vi "DAQmx Create CI Channel (sub).vi"(0 "task in":refnum<k21>, 1 "virtual channel name":string, 5 "physical channel name":tag, 7 "measurement type":i32(ring)=10125 items=["count events"=10125, "frequency"=10179, "period"=10256, "pulse width"=10359, "semi period"=10289, "pulse frequency"=15864, "pulse time"=15865, "pulse ticks"=15866, "two edge separation"=10267, "angular encoder"=10360, "linear encoder"=10361, "gps timestamp"=10362], 11 "error in":errorcluster, 13 "custom scale":tag) -> (4 "task out":refnum<k21>, 6 "channel names":string, 15 "error out":errorcluster)   [LabVIEW 2013]
uses:
  nilvaiu.dll
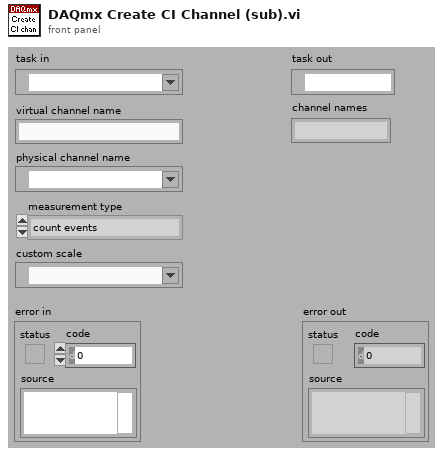
[diagram p1: front panel]
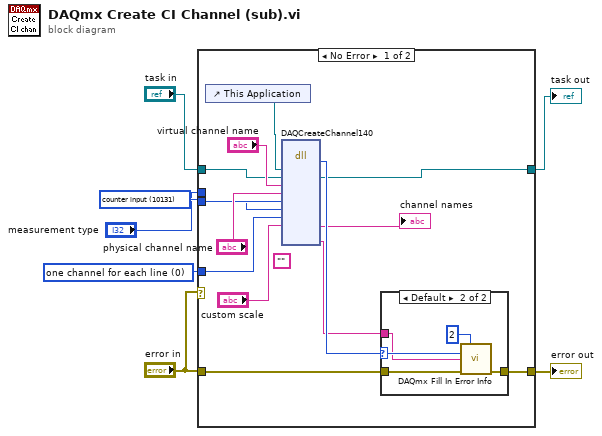
[diagram p0: block diagram]
diagram:
  w3 = 0 items=["one channel for each line", "one channel for all lines"] ("line grouping")
  w4 = 10131 items=["analog input"=10100, "analog output"=10102, "digital input"=10151, "digital output"=10153, "counter input"=10131, "counter output"=10132] ("channel type")
  n1 = case shown="No Error" "error in" {
    tunnel: [w17 w29] -> w7
    tunnel: "error in" -> [w19 w29]
    tunnel: "task in" -> [w9 w28]
    tunnel: "measurement type" -> [w16 _]
    tunnel: w4 -> [w15 _]
    tunnel: w3 -> [w11 _]
    tunnel: [w10 w28] -> w1
    frame No Error {
      (unwired) ""
      n2 = control-ref of="This Application"() -> (w8:refnum<vi>)
      n3 = dll-call lib="nilvaiu.*" fn="DAQCreateChannel140"("lvAppReference"=w8, "taskID"=w9, "virtual chnanel name"="virtual channel name", "physical channel name"="physical channel name", "measurement type"=w16, "channel type"=w15, "line grouping"=w11, "customScale"="custom scale") -> ("return type"=w18:i32, "taskID"=w10:refnum<k21>, "channel names"=→"channel names":string, "extendedErrorIndo"=w12:string)  [unwired: 10 in, 4 out]
      n4 = case shown="Default" w18 {
        selector: w18 -> [_ w25]
        tunnel: w19 -> [w22 w27]
        tunnel: [w22 w26] -> w17
        tunnel: w12 -> [_ w24]
        frame 0 {
        }
        frame Default {
          n5 = call "DAQmx Fill In Error Info.vi"("depth"=2, "status code"=w25, "extended error info"=w24, "error in"=w27) -> ("error out"=w26:errorcluster)  [unwired: 1 in, 10 out]
        }
      }
    }
    frame Error {
    }
  }
  "error out" <- w7
  "task out" <- w1
